vi "subvi_Set_zero.vi"(8 "에러 입력(에러 없음)":errorcluster, 11 "Modbus Master 입력":refnum<class "Modbus Master.lvclass">) -> (0 "에러 출력":errorcluster, 3 "Modbus Master 출력":refnum<class "Modbus Master.lvclass">)   [LabVIEW 2016]
uses:
  <vilib>/NI/Modbus Library/API/Master/Modbus Master.lvclass
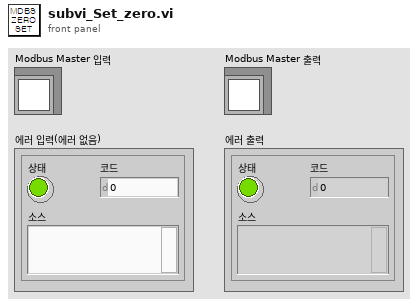
[diagram p1: front panel]
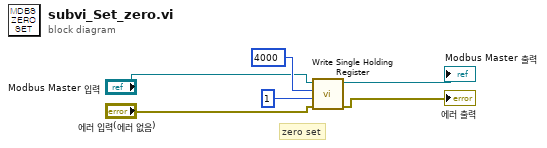
[diagram p0: block diagram]
diagram:
  # "zero set"
  n1 = call-dynamic "Write Single Holding Register.vi"("error in"="에러 입력(에러 없음)", "register to write"=u16 1, "address"=u16 4000, "Modbus master in"="Modbus Master 입력") -> ("error out"=→"에러 출력":errorcluster, "Modbus master out"=→"Modbus Master 출력":refnum<class "Modbus Master.lvclass">)  [unwired: 6 in]
